vi "Cowl_Execute.vi"() -> ()   [LabVIEW 2019]
uses:
  Cowl_Cluster.ctl
  Cowl_States.ctl
  Utility VIs/Basic_Motor_Modes.ctl
  Cowl_Globals.vi
panel:
  out "Cowl_Output":dbl
  in  "Kp":dbl
  # "e"
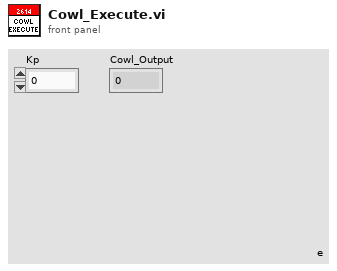
[diagram p1: front panel]
types:
  T1 = typedef "Cowl_Cluster.ctl" = cluster{"Control_State\n":T2, "Manual_Cowl_%Power":dbl}
  T2 = typedef "Cowl_States.ctl" = enum16{"Manual_%VBus", "GoToAngle"}
  T3 = typedef "Basic_Motor_Modes.ctl" = enum16{"Percent_Voltage", "Speed_Control", "Position_Control", "Current"}
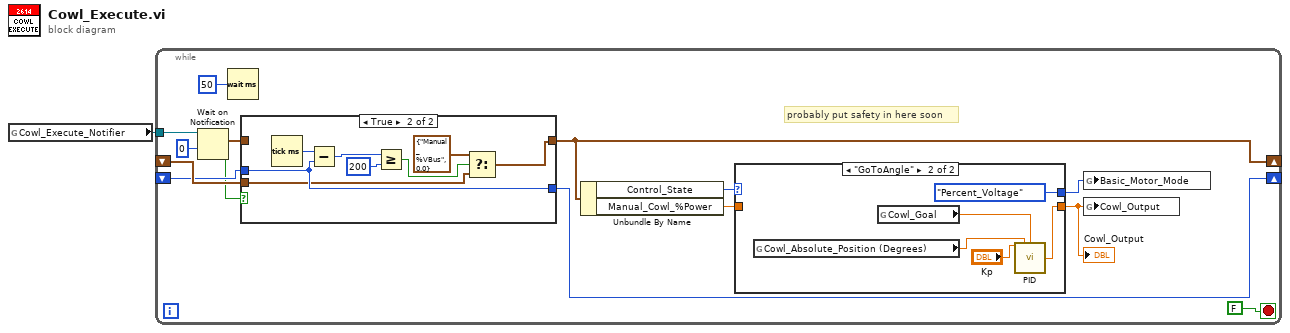
[diagram p0: block diagram]
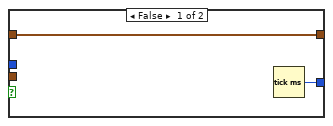
[diagram p2: hidden frame]
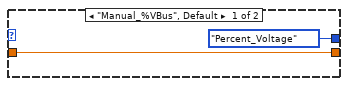
[diagram p3: hidden frame]
diagram:
  n1 = global read "Cowl_Globals.vi" "Cowl_Execute_Notifier"() -> (w1:refnum<notifier>)
  n2 = while {
    tunnel: w1 -> [w13]
    shift-right: [w5] -> _
    shift-left: _ -> [w6]
    shift-right: [w8] -> _
    shift-left: _ -> [w4]
    stop <- FALSE stop-if-true
    # "probably put safety in here soon"
    n3 = Wait on Notification(notifier=w13, timeout in ms (-1)=0) -> (notification=w7:T1, timed out?=w3:bool)  [unwired: 2 in, 2 out]
    n4 = Wait (ms)(milliseconds to wait=u32 50) -> ()  [unwired: 1 out]
    n5 = case shown="True" w3 {
      tunnel: w7 -> [w17 _]
      tunnel: [w17 w20] -> w5
      tunnel: [w16 w24] -> w8
      tunnel: w4 -> [_ w24]
      tunnel: w6 -> [_ w19]
      frame False {
        n6 = Tick Count (ms)() -> (millisecond timer value=w16:u32)
      }
      frame True {
        n7 = Tick Count (ms)() -> (millisecond timer value=w25:u32)
        n8 = Subtract(x=w25, y=w24) -> (x-y=w23:u32)
        n9 = Greater Or Equal?(x=w23, y=u32 200) -> (x >= y?=w21:bool)
        n10 = Select(t=T1 {"Control_State\n"=enum."Manual_%VBus", "Manual_Cowl_%Power"=0.0} ("notification"), s=w21, f=w19) -> (s? t:f=w20:T1)
      }
    }
    n11 = Unbundle By Name(w5) -> ("Control_State"=w12:T2, "Manual_Cowl_%Power"=w11:dbl)
    n12 = case shown="\"GoToAngle\"" w12 {
      tunnel: w11 -> [w27 _]
      tunnel: [w27 w32] -> w10
      tunnel: [Basic_Motor_Modes."Percent_Voltage" ("Basic_Motor_Mode") Basic_Motor_Modes."Percent_Voltage" ("Basic_Motor_Mode")] -> w9
      frame "Manual_%VBus", Default {
      }
      frame "GoToAngle" {
        n13 = global read "Cowl_Globals.vi" "Cowl_Absolute_Position (Degrees)"() -> (w29:dbl)
        n14 = global read "Cowl_Globals.vi" "Cowl_Goal"() -> (w30:dbl)
        n15 = call "PID.vi"("Kp"="Kp", "Process Variable"=w29, "Goal"=w30) -> ("Command"=w32:dbl)  [unwired: 10 in, 2 out]
      }
    }
    "Cowl_Output" <- w10
    n16 = global write "Cowl_Globals.vi" "Basic_Motor_Mode"(w9) -> ()
    n17 = global write "Cowl_Globals.vi" "Cowl_Output"(w10) -> ()
  }
